vi "Watchdog.vi"(8 "error in (no error)":errorcluster, 11 "IED in":refnum<class "IED.lvclass">) -> (0 "error out":errorcluster, 3 "IED out":refnum<class "IED.lvclass">)   [LabVIEW 2015, in "IED Actor.lvlib" / "IED.lvclass"]
uses:
  IED.lvclass
  Watchdog Actor/Watchdog/Watchdog.lvclass
  IED.lvclass/IED.ctl
  <vilib>/ActorFramework/Actor/Actor.lvclass
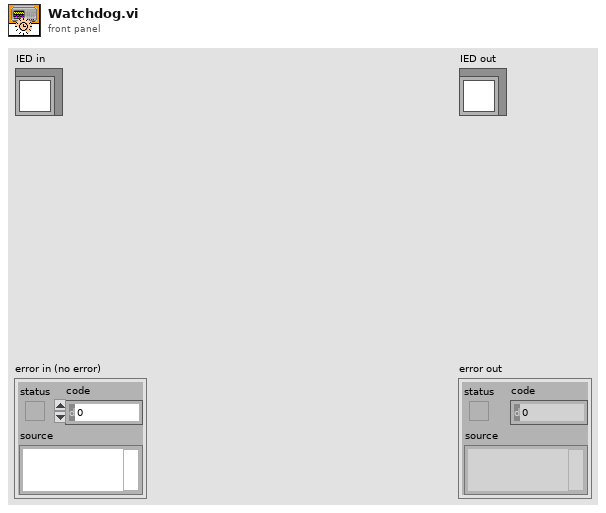
[diagram p1: front panel]
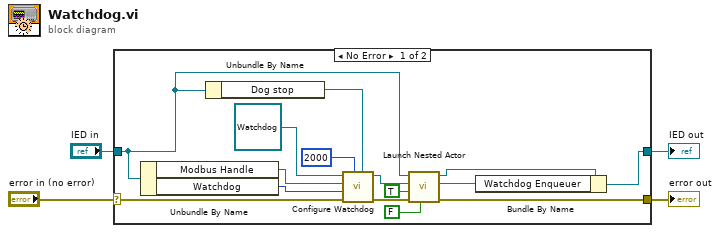
[diagram p0: block diagram]
diagram:
  n1 = case shown="No Error" "error in (no error)" {
    selector: "error in (no error)" -> [w18 w21]
    tunnel: [w14 w21] -> w3
    tunnel: [w12 w20] -> w1
    tunnel: "IED in" -> [w8 w20]
    frame No Error {
      n2 = Unbundle By Name(w8) -> ("Modbus Handle"=w10:refnum<class "Modbus Master.lvclass">, "Watchdog"=w9:u16)
      n3 = Unbundle By Name(w8) -> ("Dog stop"=w7:refnum<notifier>)
      n4 = call "Configure Watchdog.vi"("Dog stop notifier"=w7, "Period"=2000, "error in (no error)"=w18, "Register"=w9, "Modbus Handle"=w10, "Watchdog in"=refnum<class "Watchdog.lvclass"> refnum ("Watchdog Actor.lvlib:Watchdog.lvclass")) -> ("error out"=w15:errorcluster, "Watchdog out"=w13:refnum<class "Watchdog.lvclass">)  [unwired: 4 in]
      n5 = call <vilib>:"Launch Nested Actor.vi"("Open Actor Core front panel? (F)"=FALSE, "error in (no error)"=w15, "Auto-stop? (T)"=TRUE, "Nested Actor"=w13, "Caller Actor in"=w8) -> ("error out"=w14:errorcluster, "Nested Actor's Enqueuer"=w11:refnum<class "Message Enqueuer.lvclass">, "Caller Actor out"=w16:refnum<class "IED.lvclass">)  [unwired: 4 in]
      n6 = Bundle By Name(cluster=w16, "Watchdog Enqueuer"=w11) -> (w12:refnum<class "IED.lvclass">)
    }
    frame Error {
    }
  }
  "error out" <- w3
  "IED out" <- w1
